vi "utility_edit_device_tree_items_01_01.vi"() -> ()   [LabVIEW 2015]
panel:
  in  "Device Tree":string[](tree)=["FCXF-X-03-S05"] caption="设备列表"
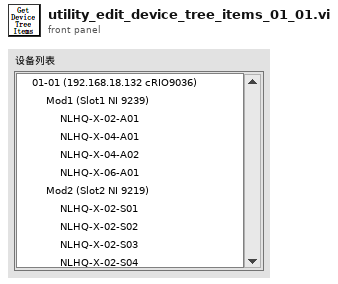
[diagram p1: front panel]
types:
  T1 = enum16{"open", "replace", "create", "open or create", "replace or create", "replace or create with confirmation"}
  T2 = cluster{"Left Cell String":string, "Child Text":string[], "Child Tag":string, "Item Indent":i32, "Child Only?":bool, "Glyph Index":i32}
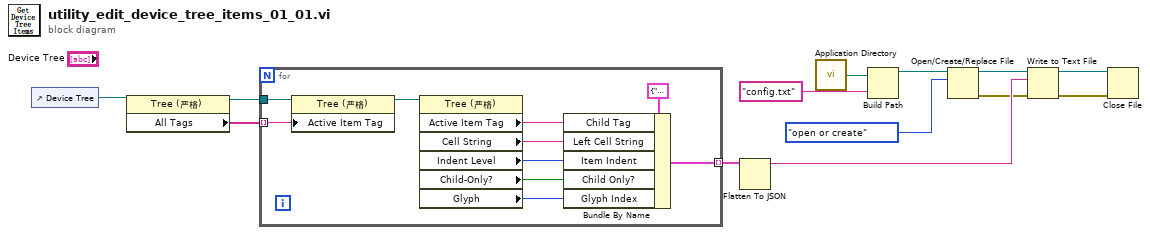
[diagram p0: block diagram]
diagram:
  n1 = control-ref of="Device Tree"() -> (w11:refnum<vi>)
  n2 = property class="Tree (严格)"(reference=w11) -> (reference out=w13:refnum<vi>, "All Tags"=w12:string[])  [unwired: 1 in, 1 out]
  n3 = for {
    tunnel: w13 -> [w23]
    tunnel: w12 -> [w21] mode=indexing
    tunnel: [w14] -> w1 mode=indexing
    n4 = property class="Tree (严格)"(reference=w23, "Active Item Tag"=w21) -> (reference out=w22:refnum<vi>)  [unwired: 1 in, 1 out]
    n5 = property class="Tree (严格)"(reference=w22) -> ("Active Item Tag"=w19:string, "Cell String"=w18:string, "Indent Level"=w17:i32, "Child-Only?"=w16:bool, "Glyph"=w15:i32)  [unwired: 1 in, 2 out]
    n6 = Bundle By Name(cluster=T2 {"Left Cell String"="FCXF-X-03-T02", "Child Text"=[], "Child Tag"="FCXF-X-03-T02", "Item Indent"=2, "Child Only?"=TRUE, "Glyph Index"=4} ("Item"), "Child Tag"=w19, "Left Cell String"=w18, "Item Indent"=w17, "Child Only?"=w16, "Glyph Index"=w15) -> (w14:T2)
  }
  n7 = Flatten To JSON(anything=w1) -> (JSON string=w10:string)  [unwired: 2 in, 1 out]
  n8 = call <vilib>:"Application Directory.vi"() -> ("Application Directory"=w5:path)
  n9 = Build Path(base path=w5, name or relative path="config.txt" ("名称或相对路径")) -> (appended path=w3:path)
  n10 = Open/Create/Replace File(file path (use dialog)=w3, operation (0:open)=T1."open or create" ("操作(0:open)")) -> (refnum out=w9:refnum<file>, error out=w7:errorcluster)  [unwired: 4 in, 1 out]
  n11 = Write to Text File(file (use dialog)=w9, text=w10, error in=w7) -> (refnum out=w8:refnum<file>, error out=w6:errorcluster)  [unwired: 1 in, 1 out]
  n12 = Close File(refnum=w8, error in=w6) -> ()  [unwired: 2 out]
